vi "Delete Last Pet.vi"(7 "Server Alias":string, 10 "Error In":errorcluster) -> (2 "Error Out":errorcluster)   [LabVIEW 2013, in "TS.lvlib"]
uses:
  TS.lvlib
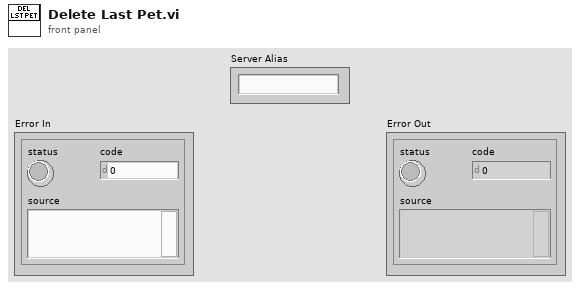
[diagram p1: front panel]
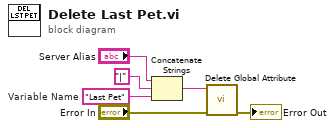
[diagram p0: block diagram]
diagram:
  w3 = "Last Pet"  # Variable Name
  n1 = Concatenate Strings("Server Alias", "|" ("string"), w3) -> (w2:string)
  n2 = call "Delete Global Attribute.vi"("Error In"="Error In", "Name"=w2) -> ("Error Out"=→"Error Out":errorcluster)  [unwired: 8 in, 1 out]
